vi "Reorder Sequence.vi"(8 "error in (no error)":errorcluster, 9 "New Index":i32, 10 "Target Step":i32, 11 "Sequence in":refnum<class "Sequence.lvclass">) -> (0 "error out":errorcluster, 3 "Sequence out":refnum<class "Sequence.lvclass">)   [LabVIEW 2024, in "Ramses Sequencer.lvlib" / "Sequence.lvclass"]
uses:
  Sequence.lvclass
  Sequence.lvclass/Sequence.ctl
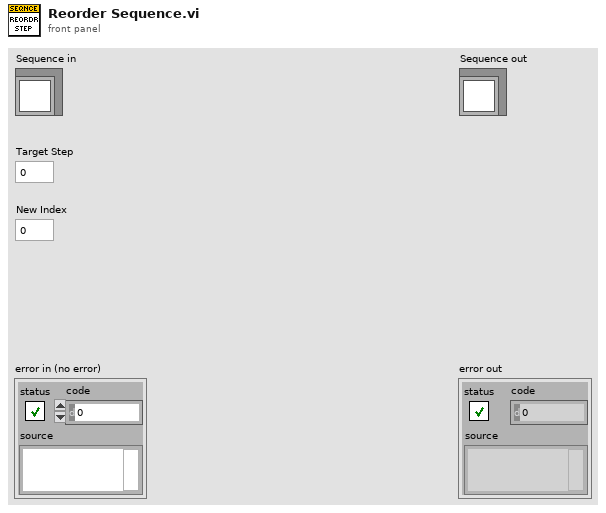
[diagram p1: front panel]
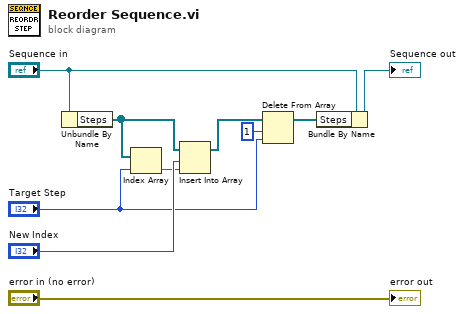
[diagram p0: block diagram]
diagram:
  n1 = Unbundle By Name("Sequence in") -> ("Steps"=w2:refnum<class "Base Step.lvclass">[])
  n2 = Index Array(array=w2, index="Target Step") -> (element=w6:refnum<class "Base Step.lvclass">)
  n3 = Insert Into Array(array=w2, index="New Index", new element=w6) -> (w1:refnum<class "Base Step.lvclass">[])
  n4 = Delete From Array(array=w1, length=1, index="Target Step") -> (array with subset deleted=w5:refnum<class "Base Step.lvclass">[])  [unwired: 1 out]
  n5 = Bundle By Name(cluster="Sequence in", "Steps"=w5) -> (→"Sequence out":refnum<class "Sequence.lvclass">)
  "error out" <- "error in (no error)"
